vi "dvp Vi Get Noise Reduct2d State.vi"(10 "pNoiseReduct2dState":i32, 11 "handle":u32) -> (2 "pNoiseReduct2dState out":i32, 3 "function return":u32(ring))   [LabVIEW 2018, in "LabViewDVPCamera.lvlib"]
doc: "LabviewDvp2Api dvpStatus dvpViGetNoiseReduct2dState(dvpHandle handle, BOOL *pNoiseReduct2dState);"
uses:
  LabViewDVPCamera.lvlib
  LabViewDVPCamera/LabViewDVPCamera.dll
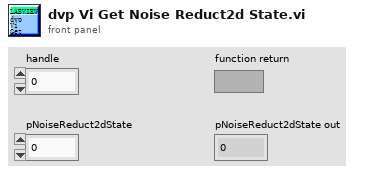
[diagram p1: front panel]
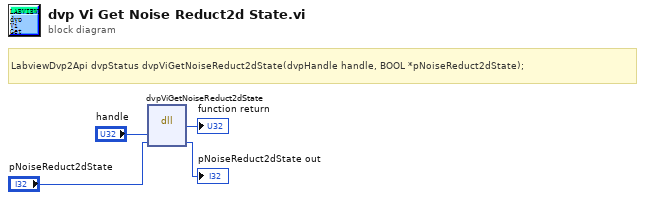
[diagram p0: block diagram]
diagram:
  # "LabviewDvp2Api dvpStatus dvpViGetNoiseReduct2dState(dvpHandle handle, BOOL *pNoiseReduct2dState);"
  n1 = dll-call lib="C:/Program Files (x86)/DVP2 Labview cn 64/Sample/LabViewDVPCamera/LabViewDVPCamera.*" fn="dvpViGetNoiseReduct2dState"("handle"="handle", "pNoiseReduct2dState"="pNoiseReduct2dState") -> (→"function return":u32, "pNoiseReduct2dState"=→"pNoiseReduct2dState out":i32)  [unwired: 4 in, 2 out]
